vi "testUnflattenTimeFromXML.vi"() -> ()   [LabVIEW 2012, in "UnitsAndXML.lvlib"]
uses:
  <userlib>/Common/UnitsAndXML/UnitsAndXML.lvlib
  <userlib>/Common/UnitsAndXML/FlattenItemWithUnitToXML/FlattenTimeToXML/TimeUnit.ctl
  <userlib>/Common/UnitsAndXML/UnflattenItemWithUnitFromXML/UnflattenTimeFromXML/typeMethods/unflattenTimeFromXML_Array.vi
  <userlib>/Common/UnitsAndXML/UnflattenItemWithUnitFromXML/UnflattenTimeFromXML/typeMethods/unflattenTimeFromXML_Scalar.vi
panel:
  out "error out":errorcluster
  out "time":dbl[unit][](array[numeric])
  out "time":dbl[unit]
  in  "timeUnitInXML":T1
  in  "xmlStringArray":string="<time>15</time>\r\n<time>30</time>\r\n<time>45</time>\r\n<time>60</time>"
  in  "xmlStringScalar":string="<time>15</time>"
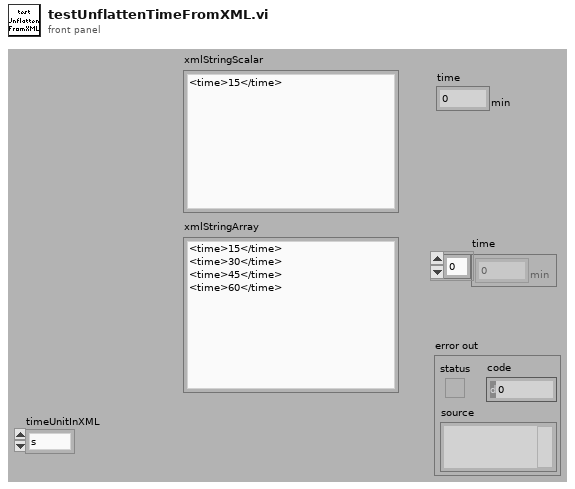
[diagram p1: front panel]
types:
  T1 = typedef "UnitsAndXML.lvlib/TimeUnit.ctl" = enum16{"s", "d", "h", "min", "a"}
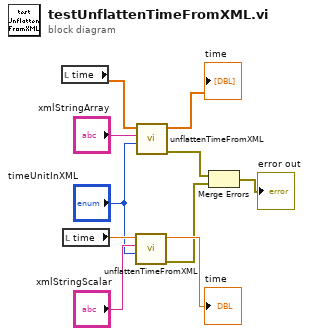
[diagram p0: block diagram]
diagram:
  n1 = local read "time"() -> (w3:dbl[unit][])
  n2 = local read "time"() -> (w9:dbl[unit])
  n3 = call-poly <userlib>:"unflattenTimeFromXML.vi"("timeUnitInXML"="timeUnitInXML", "xmlString"="xmlStringScalar", "timeForType"=w9) -> ("error out"=w5:errorcluster, "time"=→"time":dbl[unit])  [unwired: 7 in]
  n4 = call-poly <userlib>:"unflattenTimeFromXML.vi"("timeUnitInXML"="timeUnitInXML", "xmlString"="xmlStringArray", "timeForType"=w3) -> ("error out"=w6:errorcluster, "time"=→"time":dbl[unit][])  [unwired: 7 in]
  n5 = Merge Errors(w6, w5) -> (→"error out":errorcluster)
